vi "http get action.vi"(7 "transmit queue":refnum<queue>, 11 "application request in":T1) -> (0 "connection error":errorcluster)   [LabVIEW 2013, in "http responder.lvclass"]
uses:
  http responder.lvclass
  http request.ctl
  http method.ctl
  http response.ctl
  http response packet type.ctl
panel:
  in  "other":string
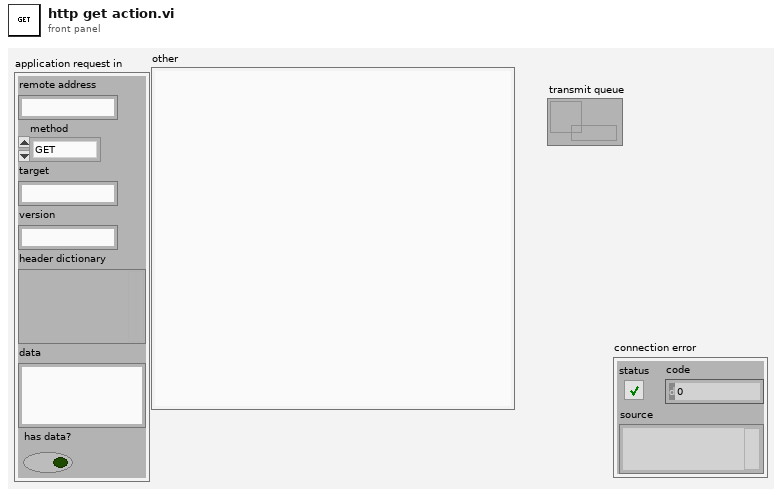
[diagram p1: front panel]
types:
  T1 = typedef "http request.ctl" = cluster{"remote address":string, "method":T2, "target":string, "version":string, "header dictionary":variant, "data":string, "has data?":bool}
  T2 = typedef "http method.ctl" = enum16{"GET", "POST", "PUT", "DELETE", "HEAD", "OPTIONS", "upgrade"}
  T3 = typedef "http response packet type.ctl" = enum16{"full response", "header only", "data only", "last data"}
  T4 = typedef "http response.ctl" = cluster{"packet type":T3, "reason code":u16, "status string":string, "header dictionary":variant, "cookies":string[], "data":string}
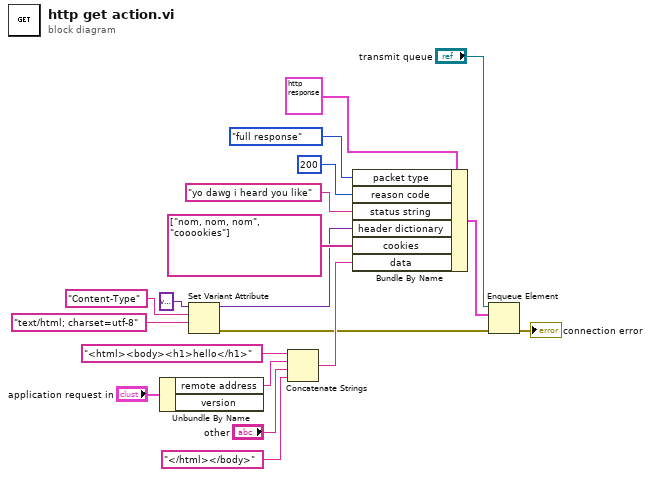
[diagram p0: block diagram]
diagram:
  n1 = Unbundle By Name("application request in") -> ("remote address"=w8:string)  [unwired: 1 out]
  n2 = Set Variant Attribute(Variant=variant ("variant"), name="Content-Type", value="text/html; charset=utf-8" ("name")) -> (Variant out=w2:variant, error out=w5:errorcluster)  [unwired: 1 in, 1 out]
  n3 = Concatenate Strings("<html><body><h1>hello</h1>" ("string"), w8, "other", "</html></body>" ("string")) -> (w9:string)
  n4 = Bundle By Name(cluster=T4 {"packet type"=enum."full response", "reason code"=0, "status string"="", "header dictionary"=variant, "cookies"=[], "data"=""} ("application request"), "packet type"=http_response_packet_type."full response", "reason code"=u16 200, "status string"="yo dawg i heard you like", "header dictionary"=w2, "cookies"=string[] ["nom, nom, nom", "cooookies"], "data"=w9) -> (w3:T4)
  n5 = Enqueue Element(queue="transmit queue", element=w3, error in (no error)=w5) -> (error out=→"connection error":errorcluster)  [unwired: 1 in, 2 out]
